vi "Example_chartsheet.vi"() -> ()   [LabVIEW 2015]
uses:
  Controls/Chart type.ctl
  Controls/lxw_chart_marker_type.ctl
  Controls/lxw_chart_legend_position.ctl
  xlsxwriter.lvlib
panel:
  out "function return 2":string
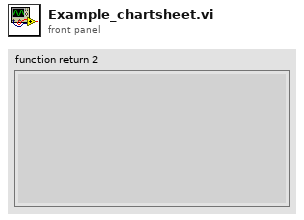
[diagram p1: front panel]
types:
  T1 = enum32{"invalid app kind", "Development System", "Run Time System", "Student Edition", "Embedded LabVIEW", "Evaluation", "Custom"}
  T2 = cluster{"color":u32, "none":u8, "@dummy control@":i8, "@dummy control@":i8, "@dummy control@":i8, "width":sgl, "dash_type":u8, "transparency":u8}
  T3 = cluster{"color":u32, "none":u8, "transparency":u8}
  T4 = typedef "lxw_chart_legend_position.ctl" = u8
  T5 = typedef "lxw_chart_marker_type.ctl" = u8
  T6 = typedef "Chart type.ctl" = u8
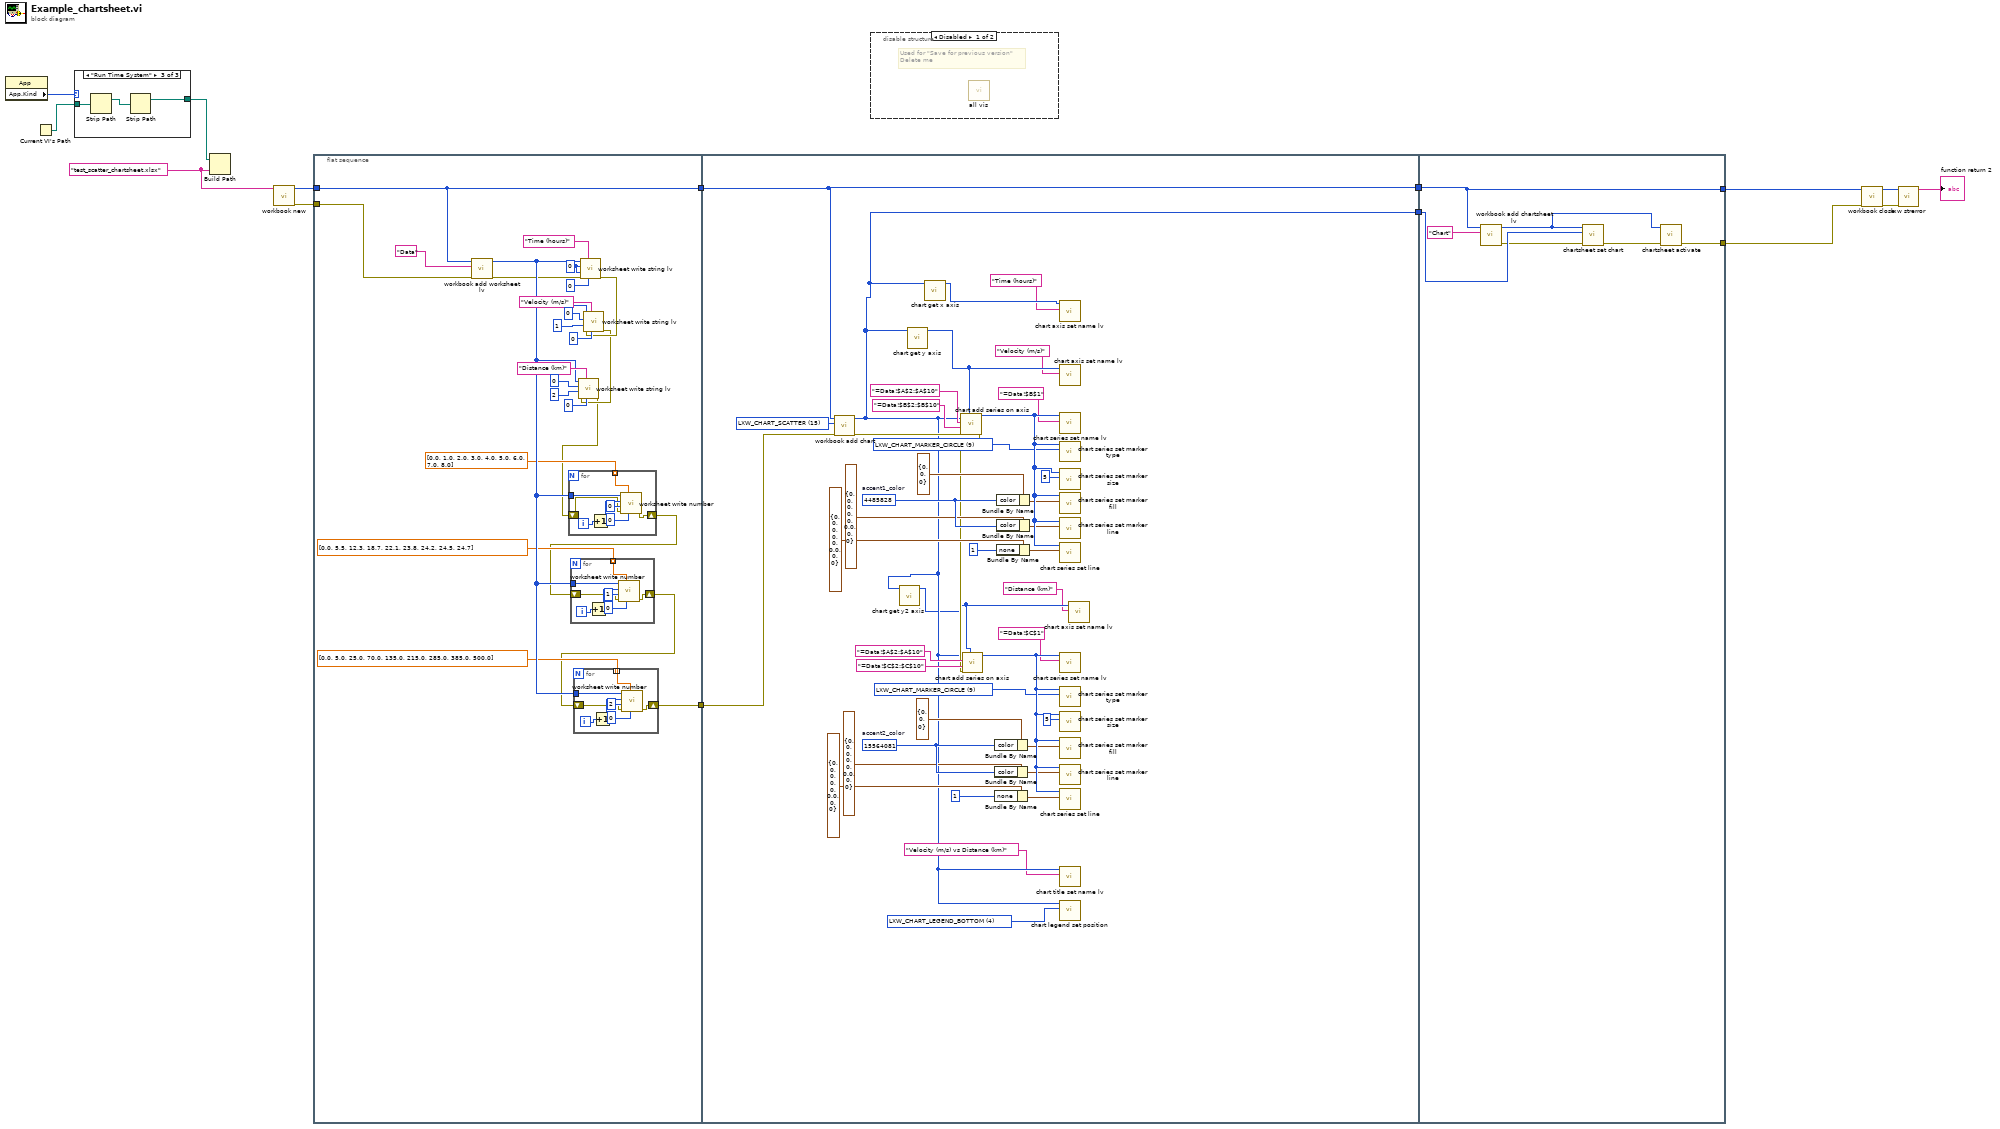
[diagram p0: block diagram]
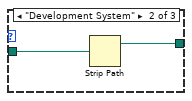
[diagram p4: hidden frame]
diagram:
  w9 = "test_scatter_chartsheet.xlsx" ("filename")
  n1 = property class="App"() -> ("App.Kind"=w14:T1)  [unwired: 2 in, 2 out]
  n2 = Current VI's Path() -> (path=w13:path)
  n3 = case shown="\"Run Time System\"" w14 {
    tunnel: w13 -> [w16 w18 w21]
    tunnel: [w16 w17 w19] -> w12
    frame "invalid app kind", Default {
    }
    frame "Development System" {
      n4 = Strip Path(path=w18) -> (stripped path=w17:path)  [unwired: 1 out]
    }
    frame "Run Time System" {
      n5 = Strip Path(path=w21) -> (stripped path=w20:path)  [unwired: 1 out]
      n6 = Strip Path(path=w20) -> (stripped path=w19:path)  [unwired: 1 out]
    }
  }
  n7 = Build Path(base path=w12, name or relative path=w9) -> ()  [unwired: 1 out]
  n8 = call "workbook new.vi"("filename"=w9) -> ("error out"=w8:errorcluster, "function return"=w15:u32)  [unwired: 9 in]
  n9 = flat-sequence {
    tunnel: w15 -> [w24]
    tunnel: w8 -> [w23]
    tunnel: [w25] -> w7
    tunnel: [w24] -> w6
    tunnel: w7 -> [w90]
    tunnel: w6 -> [w91]
    tunnel: [w91] -> w4
    tunnel: [w75] -> w3
    tunnel: [w118] -> w5
    tunnel: w4 -> [w116]
    tunnel: w3 -> [w117]
    tunnel: [w116] -> w2
    frame #0 {
      w45 = u32 0 ("row")
      n10 = call "workbook add worksheet lv.vi"("error in (no error)"=w23, "sheetname"="Data", "workbook"=w24) -> ("error out"=w22:errorcluster, "function return"=w34:u32)  [unwired: 7 in]
      n11 = call "worksheet write string lv.vi"("format"=u32 0, "string"="Time (hours)", "error in (no error)"=w22, "col"=w45, "row"=w45, "worksheet"=w34) -> ("error out"=w30:errorcluster)  [unwired: 4 in, 1 out]
      n12 = call "worksheet write string lv.vi"("format"=u32 0, "string"="Velocity (m/s)", "error in (no error)"=w30, "col"=u16 1, "row"=u32 0, "worksheet"=w34) -> ("error out"=w29:errorcluster)  [unwired: 4 in, 1 out]
      n13 = call "worksheet write string lv.vi"("format"=u32 0, "string"="Distance (km)", "error in (no error)"=w29, "col"=u16 2, "row"=u32 0, "worksheet"=w34) -> ("error out"=w28:errorcluster)  [unwired: 4 in, 1 out]
      n14 = for {
        tunnel: w34 -> [w70]
        tunnel: dbl[] [0.0, 1.0, 2.0, 3.0, 4.0, 5.0, 6.0, 7.0, 8.0] -> [w69] mode=indexing
        shift-right: [w63] -> w27
        shift-left: w28 -> [w64]
        i -> [w68]
        n15 = Increment(x=w68) -> (x+1=w67:i32)
        n16 = call "worksheet write number.vi"("format"=u32 0, "number"=w69, "error in (no error)"=w64, "col"=u16 0, "row"=w67, "worksheet"=w70) -> ("error out"=w63:errorcluster)  [unwired: 4 in, 1 out]
      }
      n17 = for {
        tunnel: w34 -> [w62]
        tunnel: dbl[] [0.0, 5.5, 12.3, 18.7, 22.1, 23.8, 24.2, 24.5, 24.7] -> [w61] mode=indexing
        shift-right: [w55] -> w26
        shift-left: w27 -> [w56]
        i -> [w60]
        n18 = Increment(x=w60) -> (x+1=w59:i32)
        n19 = call "worksheet write number.vi"("format"=u32 0, "number"=w61, "error in (no error)"=w56, "col"=u16 1, "row"=w59, "worksheet"=w62) -> ("error out"=w55:errorcluster)  [unwired: 4 in, 1 out]
      }
      n20 = for {
        tunnel: w34 -> [w54]
        tunnel: dbl[] [0.0, 5.0, 25.0, 70.0, 135.0, 215.0, 285.0, 385.0, 500.0] -> [w53] mode=indexing
        shift-right: [w47] -> w25
        shift-left: w26 -> [w48]
        i -> [w52]
        n21 = Increment(x=w52) -> (x+1=w51:i32)
        n22 = call "worksheet write number.vi"("format"=u32 0, "number"=w53, "error in (no error)"=w48, "col"=u16 2, "row"=w51, "worksheet"=w54) -> ("error out"=w47:errorcluster)  [unwired: 4 in, 1 out]
      }
    }
    frame #1 {
      w71 = T4 4 items=["LXW_CHART_LEGEND_NONE", "LXW_CHART_LEGEND_RIGHT", "LXW_CHART_LEGEND_LEFT", "LXW_CHART_LEGEND_TOP", "LXW_CHART_LEGEND_BOTTOM", "LXW_CHART_LEGEND_TOP_RIGHT", "LXW_CHART_LEGEND_OVERLAY_RIGHT", "LXW_CHART_LEGEND_OVERLAY_LEFT"] ("position")
      w99 = T5 9 items=["LXW_CHART_MARKER_AUTOMATIC", "LXW_CHART_MARKER_NONE", "LXW_CHART_MARKER_SQUARE", "LXW_CHART_MARKER_DIAMOND", "LXW_CHART_MARKER_TRIANGLE", "LXW_CHART_MARKER_X", "LXW_CHART_MARKER_STAR", "LXW_CHART_MARKER_SHORT_DASH", "LXW_CHART_MARKER_LONG_DASH", "LXW_CHART_MARKER_CIRCLE", "LXW_CHART_MARKER_PLUS"] ("type")
      w98 = T5 9 items=["LXW_CHART_MARKER_AUTOMATIC", "LXW_CHART_MARKER_NONE", "LXW_CHART_MARKER_SQUARE", "LXW_CHART_MARKER_DIAMOND", "LXW_CHART_MARKER_TRIANGLE", "LXW_CHART_MARKER_X", "LXW_CHART_MARKER_STAR", "LXW_CHART_MARKER_SHORT_DASH", "LXW_CHART_MARKER_LONG_DASH", "LXW_CHART_MARKER_CIRCLE", "LXW_CHART_MARKER_PLUS"] ("type")
      w109 = u32 15564081  # accent2_color
      w103 = u32 4485828  # accent1_color
      w92 = T6 15 items=["LXW_CHART_NONE", "LXW_CHART_AREA", "LXW_CHART_AREA_STACKED", "LXW_CHART_AREA_STACKED_PERCENT", "LXW_CHART_BAR", "LXW_CHART_BAR_STACKED", "LXW_CHART_BAR_STACKED_PERCENT", "LXW_CHART_COLUMN", "LXW_CHART_COLUMN_STACKED", "LXW_CHART_COLUMN_STACKED_PERCENT", "LXW_CHART_DOUGHNUT", "LXW_CHART_LINE", "LXW_CHART_LINE_STACKED", "LXW_CHART_LINE_STACKED_PERCENT", "LXW_CHART_PIE", "LXW_CHART_SCATTER", "LXW_CHART_SCATTER_STRAIGHT", "LXW_CHART_SCATTER_STRAIGHT_WITH_MARKERS", "LXW_CHART_SCATTER_SMOOTH", "LXW_CHART_SCATTER_SMOOTH_WITH_MARKERS", "LXW_CHART_RADAR", "LXW_CHART_RADAR_WITH_MARKERS", "LXW_CHART_RADAR_FILLED"] ("chart_type")
      n23 = call "workbook add chart.vi"("error in (no error)"=w90, "Ring"=w92, "workbook"=w91) -> ("error out"=w89:errorcluster, "function return"=w75:u32)  [unwired: 7 in]
      n24 = call "chart get y2 axis.vi"("chart"=w75) -> ("function return"=w74:u32)  [unwired: 9 in, 1 out]
      n25 = call "chart get y axis.vi"("chart"=w75) -> ("function return"=w77:u32)  [unwired: 9 in, 1 out]
      n26 = call "chart get x axis.vi"("chart"=w75) -> ("function return"=w79:u32)  [unwired: 9 in, 1 out]
      n27 = call "chart add series on axis.vi"("y_axis"=w77, "error in (no error)"=w89, "values"="=Data!$B$2:$B$10", "categories"="=Data!$A$2:$A$10", "chart"=w75) -> ("error out"=w88:errorcluster, "function return"=w112:u32)  [unwired: 5 in]
      n28 = call "chart add series on axis.vi"("y_axis"=w74, "error in (no error)"=w88, "values"="=Data!$C$2:$C$10", "categories"="=Data!$A$2:$A$10", "chart"=w75) -> ("function return"=w110:u32)  [unwired: 5 in, 1 out]
      n29 = Bundle By Name(cluster=T3 {"color"=0, "none"=0, "transparency"=0} ("fill"), "color"=w109) -> (w82:T3)
      n30 = Bundle By Name(cluster=T2 {"color"=0, "none"=0, "@dummy control@"=0, "@dummy control@"=0, "@dummy control@"=0, "width"=0.0, "dash_type"=0, "transparency"=0} ("line"), "color"=w109) -> (w80:T2)
      n31 = Bundle By Name(cluster=T2 {"color"=0, "none"=0, "@dummy control@"=0, "@dummy control@"=0, "@dummy control@"=0, "width"=0.0, "dash_type"=0, "transparency"=0} ("line"), "none"=u8 1) -> (w81:T2)
      n32 = Bundle By Name(cluster=T3 {"color"=0, "none"=0, "transparency"=0} ("fill"), "color"=w103) -> (w86:T3)
      n33 = Bundle By Name(cluster=T2 {"color"=0, "none"=0, "@dummy control@"=0, "@dummy control@"=0, "@dummy control@"=0, "width"=0.0, "dash_type"=0, "transparency"=0} ("line"), "color"=w103) -> (w85:T2)
      n34 = Bundle By Name(cluster=T2 {"color"=0, "none"=0, "@dummy control@"=0, "@dummy control@"=0, "@dummy control@"=0, "width"=0.0, "dash_type"=0, "transparency"=0} ("line"), "none"=u8 1) -> (w84:T2)
      n35 = call "chart axis set name lv.vi"("name"="Time (hours)", "axis"=w79) -> ()  [unwired: 9 in, 1 out]
      n36 = call "chart axis set name lv.vi"("name"="Velocity (m/s)", "axis"=w77) -> ()  [unwired: 9 in, 1 out]
      n37 = call "chart series set name lv.vi"("name"="=Data!$B$1", "series"=w112) -> ()  [unwired: 9 in, 1 out]
      n38 = call "chart series set marker type.vi"("type"=w98, "series"=w112) -> ()  [unwired: 9 in, 1 out]
      n39 = call "chart series set marker size.vi"("size"=u8 5, "series"=w112) -> ()  [unwired: 9 in, 1 out]
      n40 = call "chart series set marker fill.vi"("fill"=w86, "series"=w112) -> ()  [unwired: 8 in, 2 out]
      n41 = call "chart series set marker line.vi"("line"=w85, "series"=w112) -> ()  [unwired: 8 in, 2 out]
      n42 = call "chart series set line.vi"("line"=w84, "series"=w112) -> ()  [unwired: 8 in, 2 out]
      n43 = call "chart series set name lv.vi"("name"="=Data!$C$1", "series"=w110) -> ()  [unwired: 9 in, 1 out]
      n44 = call "chart series set marker type.vi"("type"=w99, "series"=w110) -> ()  [unwired: 9 in, 1 out]
      n45 = call "chart series set marker size.vi"("size"=u8 5, "series"=w110) -> ()  [unwired: 9 in, 1 out]
      n46 = call "chart series set marker fill.vi"("fill"=w82, "series"=w110) -> ()  [unwired: 8 in, 2 out]
      n47 = call "chart series set marker line.vi"("line"=w80, "series"=w110) -> ()  [unwired: 8 in, 2 out]
      n48 = call "chart series set line.vi"("line"=w81, "series"=w110) -> ()  [unwired: 8 in, 2 out]
      n49 = call "chart title set name lv.vi"("name"="Velocity (m/s) vs Distance (km)", "chart"=w75) -> ()  [unwired: 9 in, 1 out]
      n50 = call "chart legend set position.vi"("position"=w71, "chart"=w75) -> ()  [unwired: 9 in, 1 out]
      n51 = call "chart axis set name lv.vi"("name"="Distance (km)", "axis"=w74) -> ()  [unwired: 9 in, 1 out]
    }
    frame #2 {
      n52 = call "workbook add chartsheet lv.vi"("sheetname"="Chart", "workbook"=w116) -> ("error out"=w113:errorcluster, "function return"=w114:u32)  [unwired: 8 in]
      n53 = call "chartsheet set chart.vi"("error in (no error)"=w113, "chart"=w117, "chartsheet"=w114) -> ("error out"=w115:errorcluster)  [unwired: 7 in, 1 out]
      n54 = call "chartsheet activate.vi"("error in (no error)"=w115, "chartsheet"=w114) -> ("error out"=w118:errorcluster)  [unwired: 9 in]
    }
  }
  n55 = disable-structure shown="Disabled" {
    frame Disabled {
      # "Used for \"Save for previous version\"\nDelete me"
      n56 = call "all vis.vi"() -> ()  [unwired: 12 in]
    }
    frame Enabled {
    }
  }
  n57 = call "workbook close.vi"("error in (no error)"=w5, "workbook"=w2) -> ("error out"=w1:errorcluster, "function return"=w11:u32)  [unwired: 8 in]
  n58 = call "lxw strerror.vi"("error in (no error)"=w1, "error_num"=w11) -> ("function return"=→"function return 2":string)  [unwired: 8 in, 1 out]
